vi "GetWindowFlags.vi"(8 "No Error":errorcluster, 11 "Window [SDL_Window *]":i64 format="%.0x") -> (0 "Error Out":errorcluster, 3 "Window Flags":T1 items=["0"=0, "SDL_WINDOW_FULLSCREEN"=1, "SDL_WINDOW_OPENGL"=2, "SDL_WINDOW_OCCLUDED"=4, "SDL_WINDOW_HIDDEN"=8, "SDL_WINDOW_BORDERLESS"=16, "SDL_WINDOW_RESIZABLE"=32, "SDL_WINDOW_MINIMIZED"=64, "SDL_WINDOW_MAXIMIZED"=128, "SDL_WINDOW_MOUSE_GRABBED"=256, "SDL_WINDOW_INPUT_FOCUS"=512, "SDL_WINDOW_MOUSE_FOCUS"=1024, "SDL_WINDOW_EXTERNAL"=2048, "SDL_WINDOW_MODAL"=4096, "SDL_WINDOW_HIGH_PIXEL_DENSITY"=8192, "SDL_WINDOW_MOUSE_CAPTURE"=16384, "SDL_WINDOW_MOUSE_RELATIVE_MODE"=32768, "SDL_WINDOW_ALWAYS_ON_TOP"=65536, "SDL_WINDOW_UTILITY"=131072, "SDL_WINDOW_TOOLTIP"=262144, "SDL_WINDOW_POPUP_MENU"=524288, "SDL_WINDOW_KEYBOARD_GRABBED"=1048576, "SDL_WINDOW_VULKAN"=268435456, "SDL_WINDOW_METAL"=536870912, "SDL_WINDOW_TRANSPARENT"=1073741824, "SDL_WINDOW_NOT_FOCUSABLE"=2147483648])   [LabVIEW 2024, in "SDL3.lvlib" / "Video.lvlib"]
doc: "<B>Summary</B>\nGet the window flags."
uses:
  Video.lvlib
  WindowFlags--ring.ctl
  Lib/SDL3-32.dll
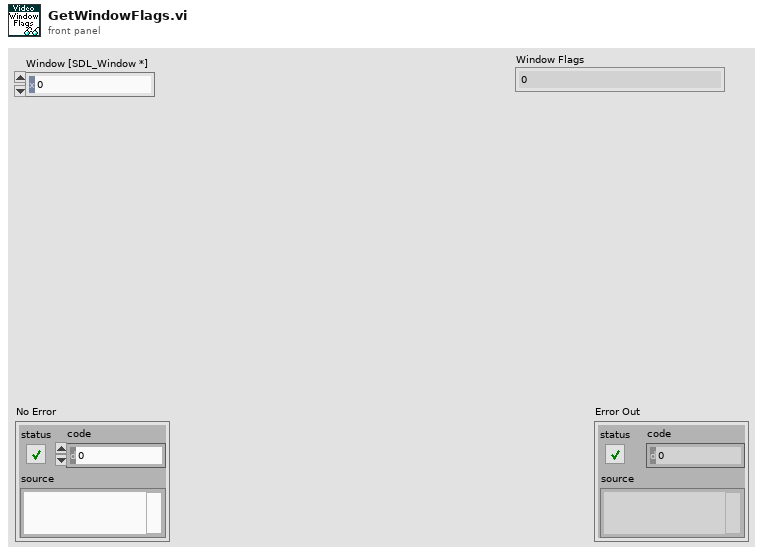
[diagram p1: front panel]
types:
  T1 = typedef "SDL3.lvlib/Video.lvlib/WindowFlags--ring.ctl" = u64
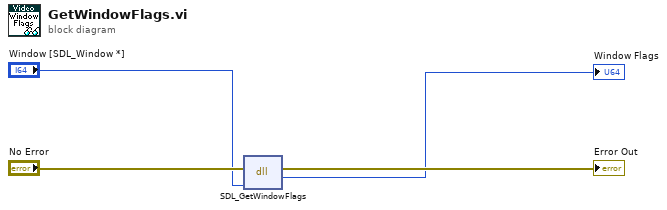
[diagram p0: block diagram]
diagram:
  n1 = dll-call lib="C:/Users/Thomas/Documents/Projects/LV-SDL3/Lib/SDL3-*.*" fn="SDL_GetWindowFlags"(error in="No Error", "window"="Window [SDL_Window *]") -> (error out=→"Error Out":errorcluster, "return type"=→"Window Flags":u64)  [unwired: 3 in, 1 out]
